vi "压力损失.vi"(0 "压力损失":sgl, 1 "压力损失判定条件":cluster{"下限":dbl, "上限":dbl}, 3 "错误输入":errorcluster) -> (8 "OK":bool, 10 "错误输出":errorcluster)   [LabVIEW 2018]
uses:
  Global_Variable/Global.vi
  Global_Variable/A180648.vi
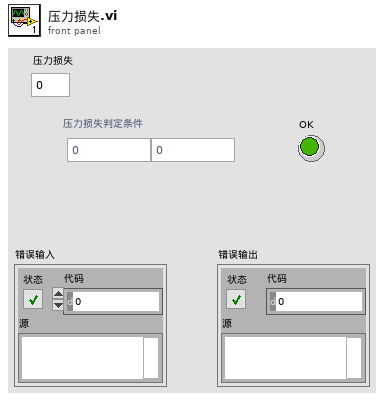
[diagram p1: front panel]
types:
  T1 = enum32{"空载", "功能", "力特性", "传感器特性", "电流特性", "振动NVH", "逆向空载", "完成"}
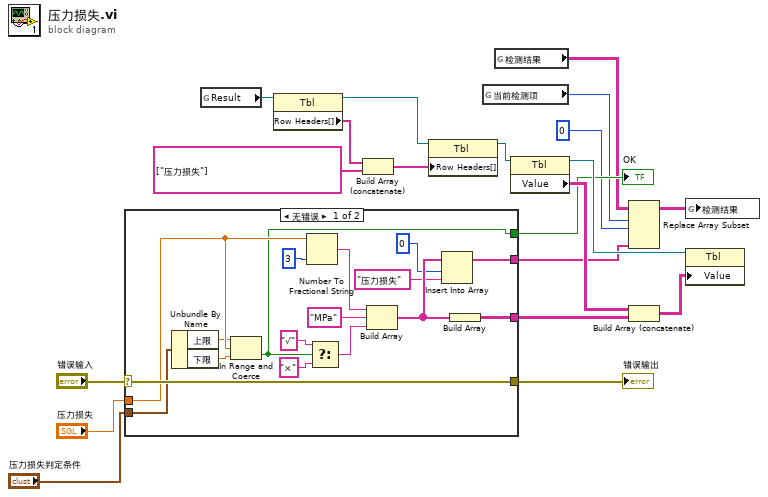
[diagram p0: block diagram]
diagram:
  n1 = case shown="无错误" "错误输入" {
    selector: "错误输入" -> [w30 w38]
    tunnel: [w30 w38] -> w19
    tunnel: [w31 _] -> w4
    tunnel: "压力损失判定条件" -> [w29 _]
    tunnel: "压力损失" -> [w28 _]
    tunnel: [w25 _] -> w8
    tunnel: [w21 _] -> w2
    frame No Error {
      n2 = Unbundle By Name(w29) -> ("上限"=w27:dbl, "下限"=w26:dbl)
      n3 = In Range and Coerce(upper limit=w27, x=w28, lower limit=w26) -> (In Range?=w25:bool)  [unwired: 1 out]
      n4 = Number To Fractional String(number=w28, precision (6)=i16 3 ("精度(6)")) -> (F-format string=w36:string)  [unwired: 2 in]
      n5 = Select(t="√", s=w25, f="×") -> (s? t:f=w32:string)
      n6 = Build Array(w36, "MPa" ("元素"), w32) -> (w24:string[])
      n7 = Insert Into Array(array=w24, index=0 ("索引"), new element="压力损失") -> (w21:string[])
      n8 = Build Array(w24) -> (w31:string[][])
    }
    frame Error {
    }
  }
  "错误输出" <- w19
  "OK" <- w8
  n9 = global read "Global.vi" "Result"() -> (w18:refnum<vi>)
  n10 = property class="Tbl"(reference=w18) -> (reference out=w15:refnum<vi>, "Row Headers[]"=w17:string[])  [unwired: 1 in, 1 out]
  n11 = Build Array (concatenate)(w17, string[] ["压力损失"] ("元素")) -> (w16:string[])
  n12 = property class="Tbl"(reference=w15, "Row Headers[]"=w16) -> (reference out=w14:refnum<vi>)  [unwired: 1 in, 1 out]
  n13 = global read "A180648.vi" "当前检测项"() -> (w6:T1)
  n14 = global read "A180648.vi" "检测结果"() -> (w7:string[][][])
  n15 = property class="Tbl"(reference=w14) -> (reference out=w13:refnum<vi>, "Value"=w12:string[][])  [unwired: 1 in, 1 out]
  n16 = Replace Array Subset(array=w7, new element=w2, index (dim 0)=w6, index (dim 1)=0 ("禁用的索引 (行)")) -> (w5:string[][][])  [unwired: 1 in]
  n17 = Build Array (concatenate)(w12, w4) -> (w11:string[][])
  n18 = global write "A180648.vi" "检测结果"(w5) -> ()
  n19 = property class="Tbl"(reference=w13, "Value"=w11) -> ()  [unwired: 1 in, 2 out]
